vi "Example_sDiscover.vi"() -> ()   [LabVIEW 2021, in "BrainStem2_LabVIEW_Library.lvlib"]
uses:
  BrainStem2_LabVIEW_Library.lvlib
panel:
  out "Array - Numeric":u32[](array[numeric])
  out "List Length":dbl
  out "sDiscover Value":dbl
  out "sDiscover Error":dbl
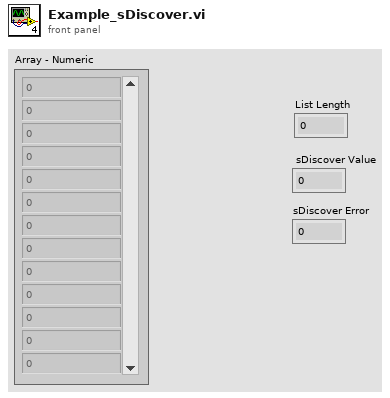
[diagram p1: front panel]
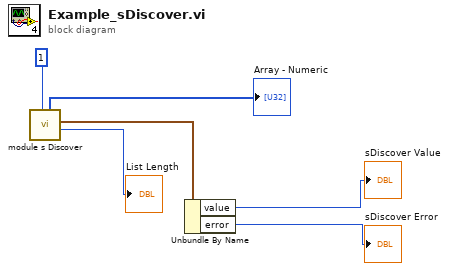
[diagram p0: block diagram]
diagram:
  n1 = call "module s Discover.vi"("transport"=1) -> ("stemListLength out"=→"List Length":i32, "result out"=w6:cluster{"value":i32, "error":i32}, "stemList"=→"Array - Numeric":u32[])  [unwired: 6 in, 2 out]
  n2 = Unbundle By Name(w6) -> ("value"=→"sDiscover Value":i32, "error"=→"sDiscover Error":i32)
